vi "_Parse SEM Result.vi"(8 "error in (no error)":errorcluster, 10 "Input String":string, 11 "VISA resource name":refnum<visa-resource-name>) -> (0 "error out":errorcluster, 1 "SEM Results":T1 {"TX Power" format="%^.3e"; "Occupied Bandwidth" format="%^.3e"}, 2 "Reliability":i32, 3 "VISA resource name out":refnum<visa-resource-name>, 5 "Out Of Tolerance":i32)   [LabVIEW 2020, in "Rohde&Schwarz CMWXP NR FR1 Measurement.lvlib"]
uses:
  <instrlib>/Rohde&Schwarz CMWXP NR FR1 Measurement/Rohde&Schwarz CMWXP NR FR1 Measurement.lvlib
  <instrlib>/Rohde&Schwarz CMWXP NR FR1 Measurement/Private/rsidr_core.llb/rsidr_core.lvlib
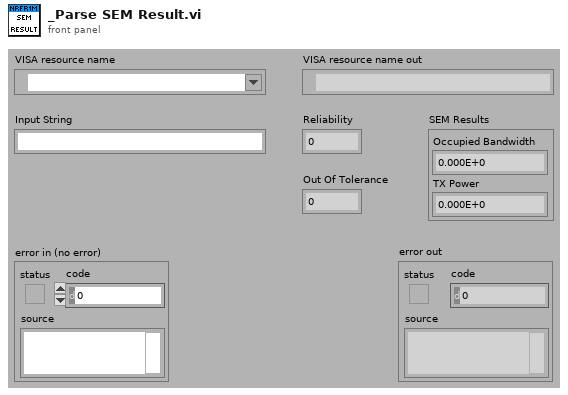
[diagram p1: front panel]
types:
  T1 = cluster{"Occupied Bandwidth":dbl, "TX Power":dbl}
  T2 = cluster{"double value out":dbl, "double value out":dbl}
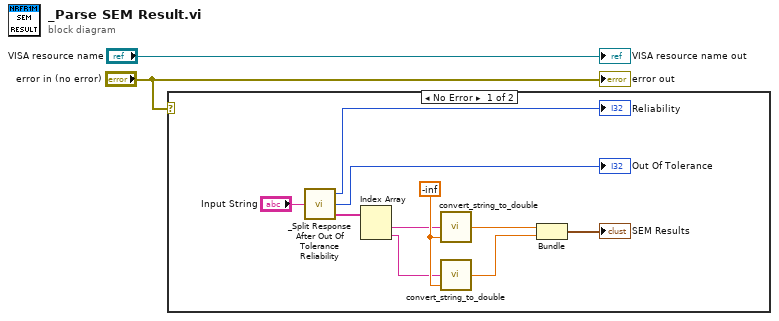
[diagram p0: block diagram]
diagram:
  n1 = case shown="No Error" "error in (no error)" {
    frame No Error {
      w12 = -inf
      n2 = call <instrlib>:"_Split Response After Out Of Tolerance Reliability.vi"("Input String"="Input String") -> ("Reliability out"=→"Reliability":i32, "Out Of Tolerance"=→"Out Of Tolerance":i32, "Response out"=w7:string[])
      n3 = Index Array(array=w7) -> (element #1=w6:string, element #2=w5:string)  [unwired: 2 in]
      n4 = call <instrlib>:"convert_string_to_double.vi"("default (0)"=w12, "String in"=w6) -> ("double value out"=w11:dbl)  [unwired: 3 in]
      n5 = call <instrlib>:"convert_string_to_double.vi"("default (0)"=w12, "String in"=w5) -> ("double value out"=w10:dbl)  [unwired: 3 in]
      n6 = Bundle("double value out"=w11, "double value out"=w10) -> (→"SEM Results":T2)  [unwired: 1 in]
    }
    frame Error {
    }
  }
  "error out" <- "error in (no error)"
  "VISA resource name out" <- "VISA resource name"
